vi "LBCB Button Label.vi"(1 "Monitor Panel":T3(ring), 2 "Rigid Connection":T1, 3 "LBCB Number":T2) -> (5 "Button Label":string)   [LabVIEW 2009]
uses:
  Data Access Objects/Metadata/LBCB Number.ctl
  Yes No Button.ctl
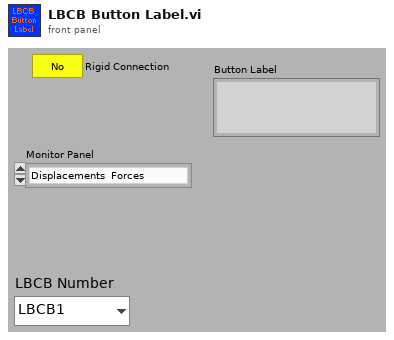
[diagram p1: front panel]
types:
  T1 = typedef "Yes No Button.ctl" = bool
  T2 = typedef "LBCB Number.ctl" = enum16{"LBCB1", "LBCB2"}
  T3 = enum32{"Displacements  Forces", "Voltages", "Mixed Mode", "Autobalance"}
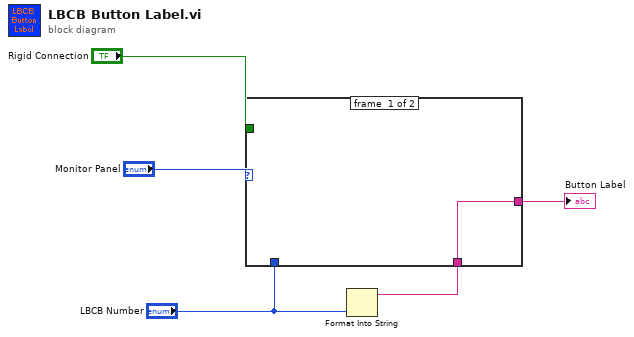
[diagram p0: block diagram]
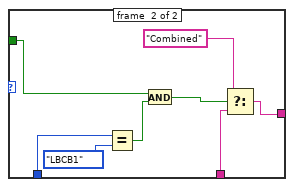
[diagram p2: hidden frame]
diagram:
  n1 = Format Into String("LBCB Number") -> (resulting string=w1:string)  [unwired: 3 in, 1 out]
  n2 = case shown="\"Mixed Mode\"" "Monitor Panel" {
    tunnel: [w6 w13] -> w4
    tunnel: w1 -> [w6 w11]
    tunnel: "Rigid Connection" -> [_ w10]
    tunnel: "LBCB Number" -> [_ w9]
    frame #0 {
    }
    frame #1 {
      n3 = Equal?(x=w9, y=LBCB_Number."LBCB1") -> (x = y?=w7:bool)
      n4 = And(x=w10, y=w7) -> (x .and. y?=w12:T1)
      n5 = Select(t="Combined", s=w12, f=w11) -> (s? t:f=w13:string)
    }
  }
  "Button Label" <- w4
